vi "datatoJson.vi"(9 "要上传的数据":string[](array[string]), 10 "数据存在则替换?":bool, 11 "上传信息输入":T1) -> (3 "utf-8 text":string)   [LabVIEW 2015]
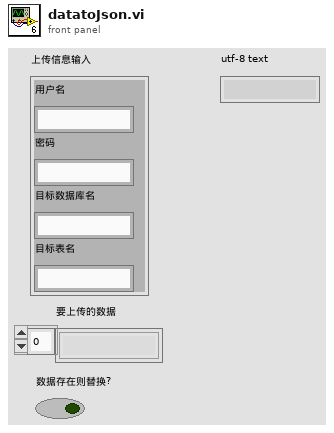
[diagram p1: front panel]
types:
  T1 = cluster{"用户名":string, "密码":string, "目标数据库名":string, "目标表名":string}
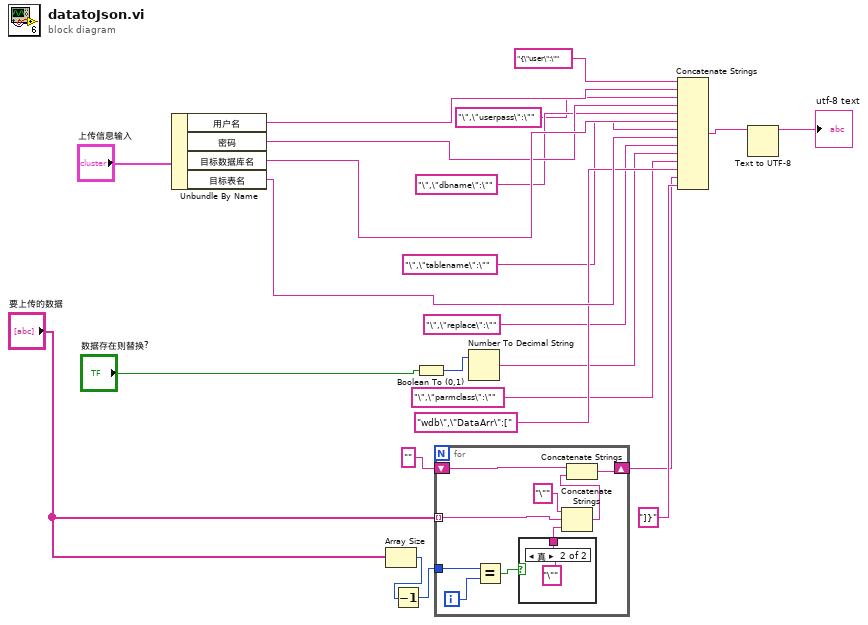
[diagram p0: block diagram]
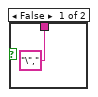
[diagram p2: hidden frame]
diagram:
  n1 = Unbundle By Name("上传信息输入") -> ("用户名"=w20:string, "密码"=w21:string, "目标数据库名"=w22:string, "目标表名"=w23:string)
  n2 = Array Size(array="要上传的数据") -> (size(s)=w14:i32)
  n3 = Decrement(x=w14) -> (x-1=w15:i32)
  n4 = Boolean To (0,1)(Boolean="数据存在则替换?") -> (0, 1=w7:i16)
  n5 = for {
    tunnel: "要上传的数据" -> [w29] mode=indexing
    shift-right: [w31] -> w12
    shift-left: "" -> [w32]
    tunnel: w15 -> [w26]
    i -> [w25]
    n6 = Equal?(x=w26, y=w25) -> (x = y?=w24:bool)
    n7 = case shown="真" w24 {
      tunnel: ["\"," ("字符串") "\"" ("字符串")] -> w28
      frame False {
      }
      frame True {
      }
    }
    n8 = Concatenate Strings("\"" ("字符串"), w29, w28) -> (w27:string)
    n9 = Concatenate Strings(w32, w27) -> (w31:string)
  }
  n10 = Number To Decimal String(number=w7) -> (decimal integer string=w8:string)  [unwired: 1 in]
  n11 = Concatenate Strings("{\"user\":\"", w20, "\",\"userpass\":\"" ("字符串"), w21, "\",\"dbname\":\"" ("字符串"), w22, "\",\"tablename\":\"" ("字符串"), w23, "\",\"replace\":\"" ("字符串"), w8, "\",\"parmclass\":\"" ("字符串"), "wdb\",\"DataArr\":[" ("字符串"), w12, "]}" ("字符串")) -> (w16:string)
  n12 = Text to UTF-8(11:w16) -> (3:→"utf-8 text":string)  [unwired: 2 in, 1 out]
